vi "guid wrap data.vi"(10 "identifier":string, 11 "data to wrap":string) -> (2 "uuid":string, 3 "wrapped data":string)   [LabVIEW 2013, in "TBM configuration.lvclass"]
doc: "Generates a packed dataset of the form\n<(additional identifier followed by a space if it is not an empty string)(randomly generated guid)>(data to wrap)</(id)(guid)>"
uses:
  TBM configuration.lvclass
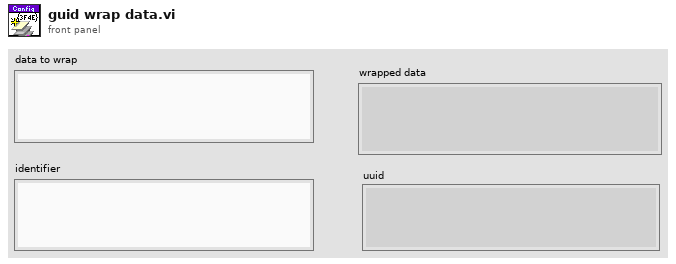
[diagram p1: front panel]
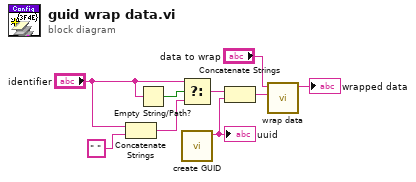
[diagram p0: block diagram]
diagram:
  n1 = Concatenate Strings("identifier", " ") -> (w6:string)
  n2 = Empty String/Path?(string/path="identifier") -> (empty?=w8:bool)
  n3 = Select(t="identifier", s=w8, f=w6) -> (s? t:f=w5:string)
  n4 = call "create GUID.vi"() -> ("uuid"=w4:string)  [unwired: 11 in]
  "uuid" <- w4
  n5 = Concatenate Strings(w5, w4) -> (w3:string)
  n6 = call "wrap data.vi"("identifier"=w3, "data to wrap"="data to wrap") -> ("wrapped data"=→"wrapped data":string)  [unwired: 9 in]
